vi "Apply Theme To UI Controls.vi"(8 "Error In":errorcluster, 11 "Appearance Actor in":refnum<class "Appearance Actor.lvclass">) -> (0 "Error Out":errorcluster, 3 "Appearance Actor out":refnum<class "Appearance Actor.lvclass">)   [LabVIEW 2021, in "Appearance Actor.lvlib" / "Appearance Actor.lvclass"]
uses:
  Appearance Actor.lvclass
  Appearance Actor.lvclass/Appearance Actor.ctl
  Theme Classes/Generic Theme/API/Typedefs/Window Element--enum.ctl
  Theme Classes/Generic Theme/Generic Theme.lvclass
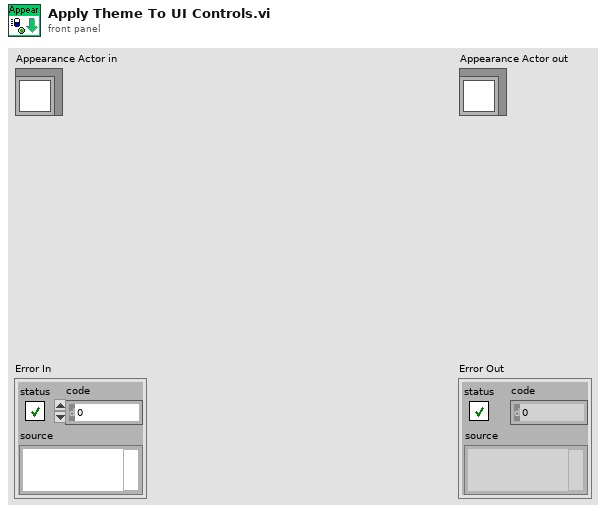
[diagram p1: front panel]
types:
  T1 = typedef "Appearance Actor.lvlib/Generic Theme.lvclass/Window Element--enum.ctl" = enum16{"None", "TB", "SM", "BP", "SB"}
  T2 = typedef "Appearance Actor.lvlib/Appearance Actor.lvclass/Control Reference Lists--cluster.ctl" = cluster{"TitleBar":T3, "SideMenu":T4, "BodyPane":T5, "StatusBar":T6}
  T3 = typedef "Appearance Actor.lvlib/Appearance Actor.lvclass/Control Reference Lists-TitleBar--cluster.ctl" = cluster{"Pane":refnum<vi>[], "Title":refnum<vi>, "Dark-CloseButton":refnum<vi>, "Light-CloseButton":refnum<vi>, "Dark-Buttons":refnum<vi>[], "Light-Buttons":refnum<vi>[], "Splitter":refnum<vi>}
  T4 = typedef "Appearance Actor.lvlib/Appearance Actor.lvclass/Control Reference Lists-SideMenu--cluster.ctl" = cluster{"Pane":refnum<vi>[], "Dark-Buttons":refnum<vi>[], "Light-Buttons":refnum<vi>[], "Splitter":refnum<vi>}
  T5 = typedef "Appearance Actor.lvlib/Appearance Actor.lvclass/Control Reference Lists-BodyPane--cluster.ctl" = cluster{"Pane":refnum<vi>[], "SubPanel":refnum<vi>}
  T6 = typedef "Appearance Actor.lvlib/Appearance Actor.lvclass/Control Reference Lists-StatusBar--cluster.ctl" = cluster{"Pane":refnum<vi>[], "Dark-Buttons":refnum<vi>[], "Light-Buttons":refnum<vi>[], "Splitter":refnum<vi>}
  T7 = typedef "Appearance Actor.lvlib/Generic Theme.lvclass/Theme Info--cluster.ctl" = cluster{"Name":string, "Type":string, "Version":string}
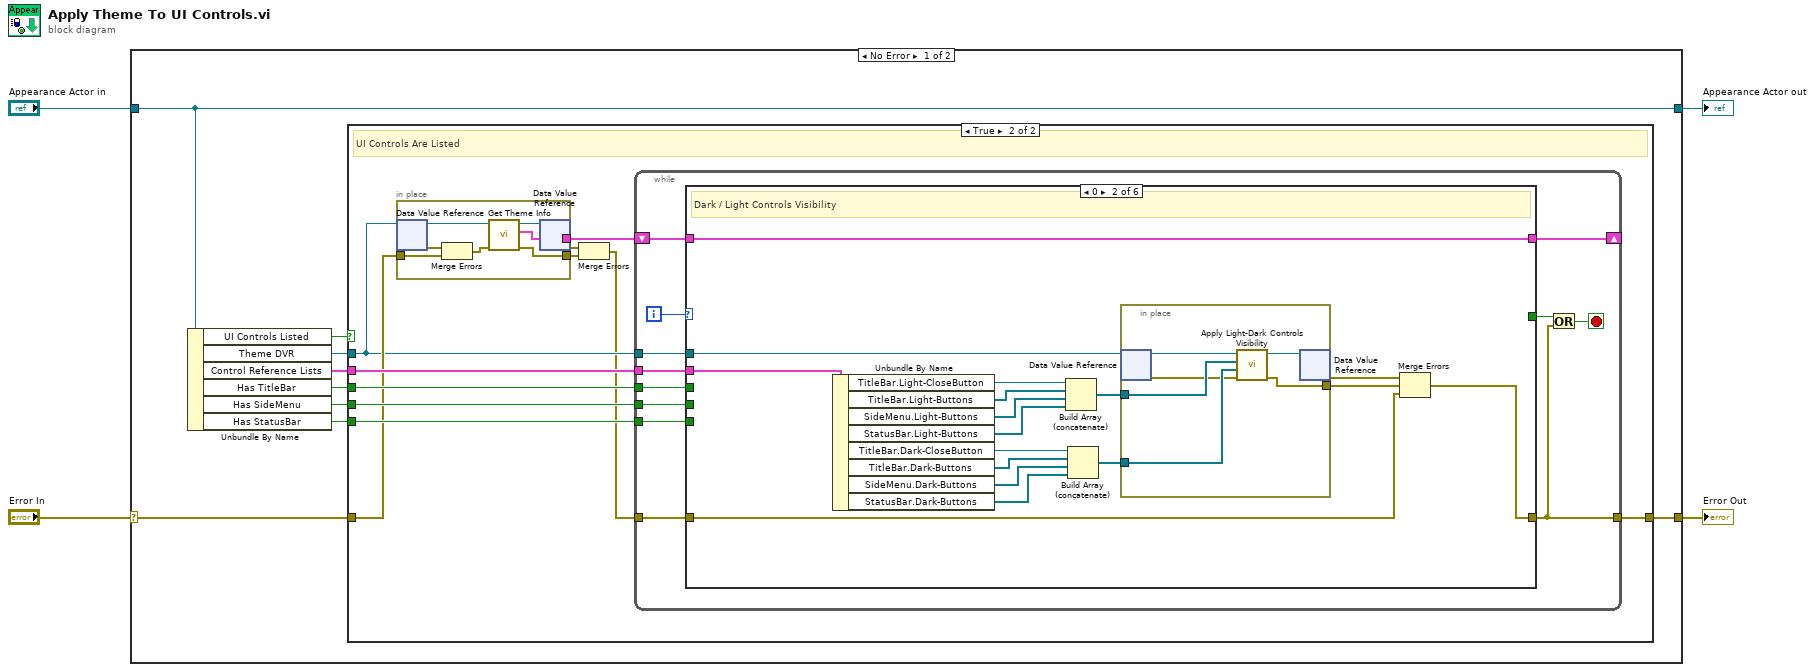
[diagram p0: block diagram]
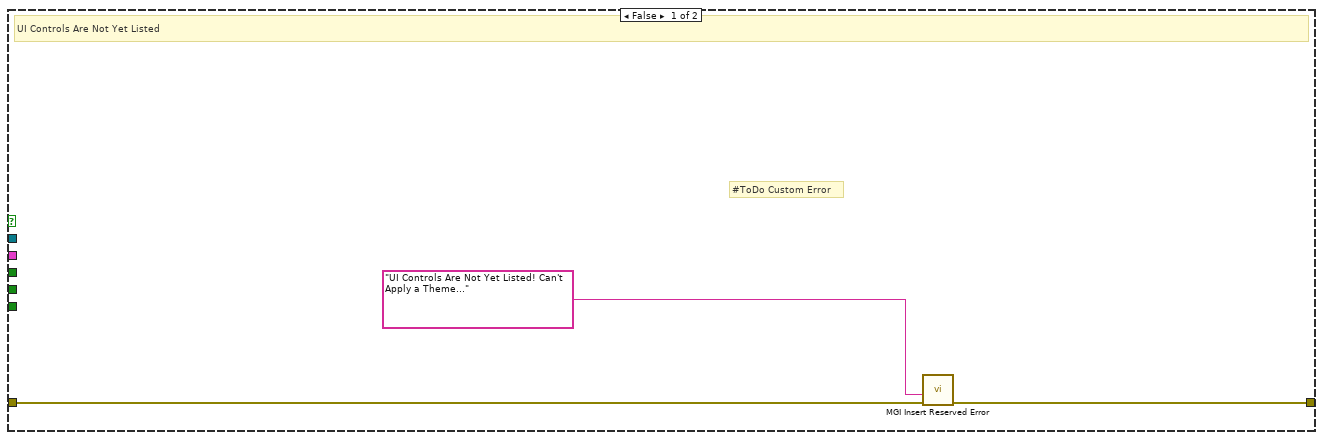
[diagram p2: hidden frame]
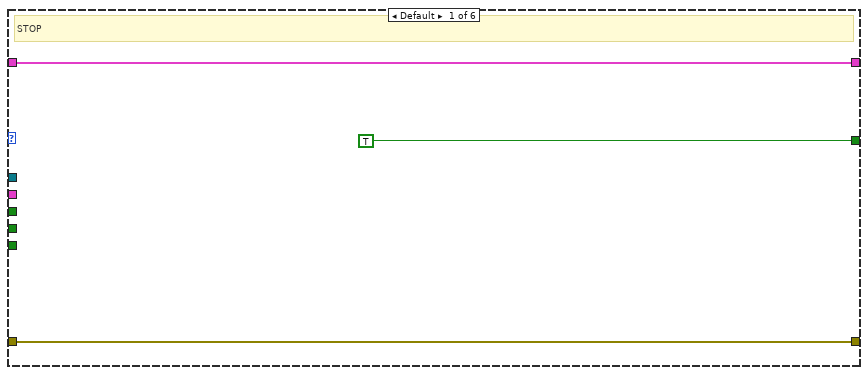
[diagram p3: hidden frame]
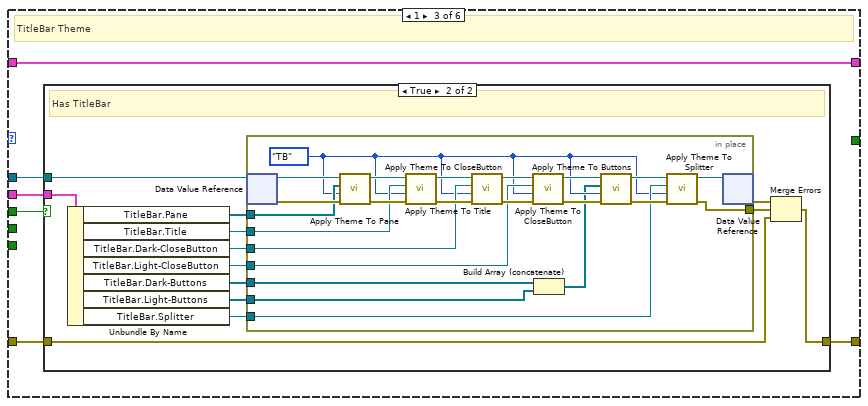
[diagram p4: hidden frame]
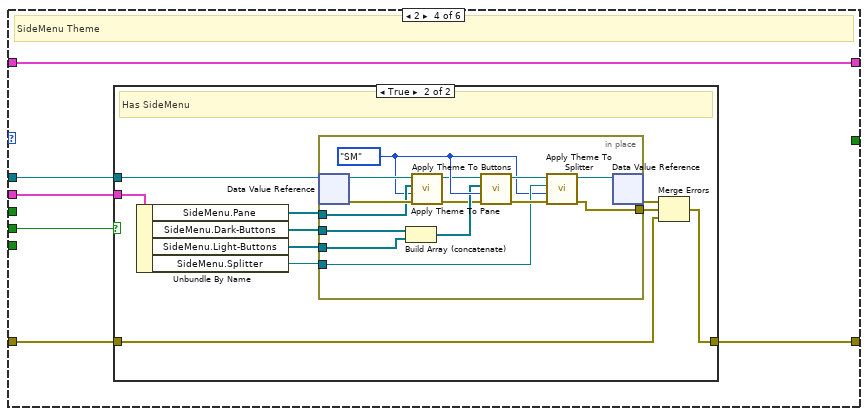
[diagram p6: hidden frame]
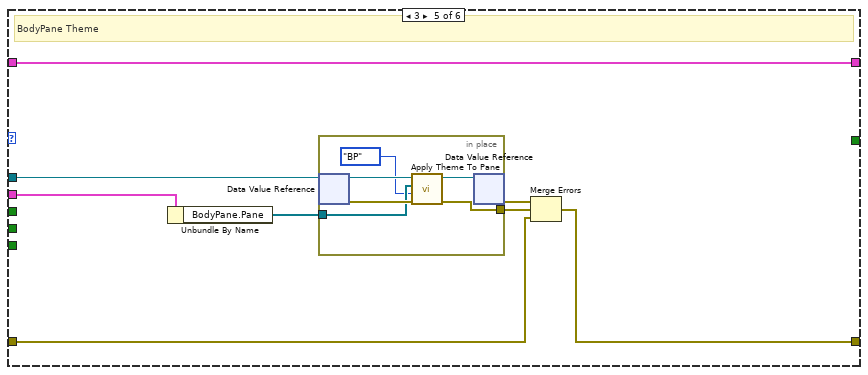
[diagram p8: hidden frame]
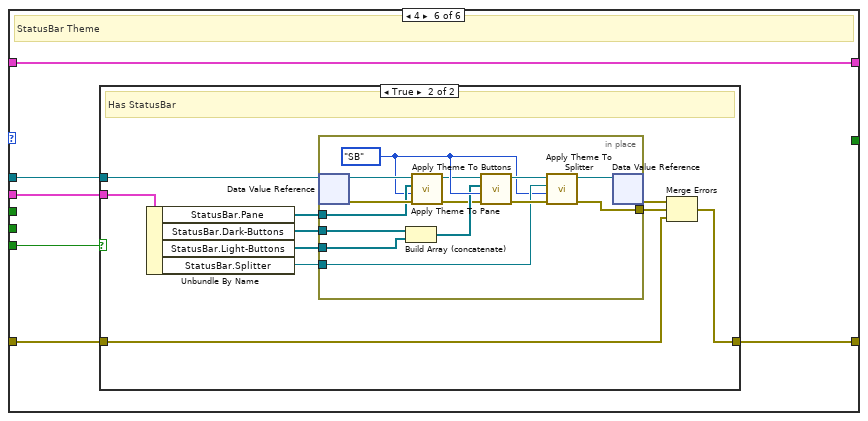
[diagram p9: hidden frame]
diagram:
  n1 = case shown="No Error" "Error In" {
    selector: "Error In" -> [w11 w193]
    tunnel: [w10 w193] -> w3
    tunnel: [w13 w192] -> w1
    tunnel: "Appearance Actor in" -> [w13 w192]
    frame No Error {
      n2 = Unbundle By Name(w13) -> ("UI Controls Listed"=w5:bool, "Theme DVR"=w12:refnum<data-value>, "Control Reference Lists"=w9:T2, "Has TitleBar"=w8:bool, "Has SideMenu"=w7:bool, "Has StatusBar"=w6:bool)
      n3 = case shown="True" w5 {
        tunnel: w12 -> [_ w20]
        tunnel: w11 -> [w16 w21]
        tunnel: [w15 w27] -> w10
        tunnel: w9 -> [_ w26]
        tunnel: w8 -> [_ w25]
        tunnel: w7 -> [_ w24]
        tunnel: w6 -> [_ w23]
        frame False {
          # "#ToDo Custom Error"
          # "UI Controls Are Not Yet Listed"
          n4 = call <userlib>:"MGI Insert Reserved Error.vi"("Error In"=w16, "Error Description"="UI Controls Are Not Yet Listed! Can't Apply a Theme..." ("format string")) -> ("Error Out"=w15:errorcluster)  [unwired: 9 in]
        }
        frame True {
          # "UI Controls Are Listed"
          n5 = in-place {
            in-place-border: [w34] -> w22
            in-place-border: w21 -> [w28]
            in-place-border: [w33] -> w17
            n6 = in-place-dvr #1(w20) -> (w32:refnum<class "Generic Theme.lvclass">, w30:errorcluster)
            n7 = Merge Errors(w30, w28) -> (w29:errorcluster)
            n8 = call-dynamic "Get Theme Info.vi"("Error In"=w29, "Generic Theme in"=w32) -> ("Error Out"=w33:errorcluster, "Theme Info"=w34:T7, "Generic Theme out"=w31:refnum<class "Generic Theme.lvclass">)  [unwired: 7 in]
            n9 = in-place-dvr #1(w31) -> (w18:errorcluster)  [unwired: 1 out]
          }
          n10 = Merge Errors(w18, w17) -> (w19:errorcluster)
          n11 = while {
            tunnel: w20 -> [w45]
            tunnel: w26 -> [w44]
            tunnel: w19 -> [w40]
            tunnel: [w41] -> w27
            tunnel: w25 -> [w39]
            tunnel: w24 -> [w38]
            tunnel: w23 -> [w37]
            shift-right: [w36] -> _
            shift-left: w22 -> [w35]
            i -> [w46]
            stop <- w42 stop-if-true
            n12 = case shown="0" w46 {
              tunnel: w45 -> [_ w52 w78 w121 w154 w166]
              tunnel: w44 -> [_ w63 w76 w118 w151 w164]
              tunnel: [TRUE _ _ _ _ _] -> w43
              tunnel: w40 -> [w48 w53 w74 w117 w148 w162]
              tunnel: [w48 w64 w77 w120 w152 w165] -> w41
              tunnel: w39 -> [_ _ w75 _ _ _]
              tunnel: w38 -> [_ _ _ w119 _ _]
              tunnel: w37 -> [_ _ _ _ _ w163]
              tunnel: [w47 w51 w73 w116 w147 w161] -> w36
              tunnel: w35 -> [w47 w51 w73 w116 w147 w161]
              frame Default {
                # "STOP"
              }
              frame 0 {
                # "Dark / Light Controls Visibility"
                n13 = Unbundle By Name(w63) -> ("TitleBar.Light-CloseButton"=w62:refnum<vi>, "TitleBar.Light-Buttons"=w61:refnum<vi>[], "SideMenu.Light-Buttons"=w60:refnum<vi>[], "StatusBar.Light-Buttons"=w59:refnum<vi>[], "TitleBar.Dark-CloseButton"=w58:refnum<vi>, "TitleBar.Dark-Buttons"=w57:refnum<vi>[], "SideMenu.Dark-Buttons"=w56:refnum<vi>[], "StatusBar.Dark-Buttons"=w55:refnum<vi>[])
                n14 = Build Array (concatenate)(w62, w61, w60, w59) -> (w50:refnum<vi>[])
                n15 = Build Array (concatenate)(w58, w57, w56, w55) -> (w54:refnum<vi>[])
                n16 = in-place {
                  in-place-border: [w71] -> w65
                  in-place-border: w50 -> [w70]
                  in-place-border: w54 -> [w69]
                  n17 = in-place-dvr #2(w52) -> (w68:refnum<class "Generic Theme.lvclass">, w67:errorcluster)
                  n18 = call-dynamic "Apply Light-Dark Controls Visibility.vi"("Error In"=w67, "Dark Controls"=w69, "Light Controls"=w70, "Generic Theme in"=w68) -> ("Error Out"=w71:errorcluster, "Generic Theme out"=w72:refnum<class "Generic Theme.lvclass">)  [unwired: 6 in]
                  n19 = in-place-dvr #2(w72) -> (w66:errorcluster)  [unwired: 1 out]
                }
                n20 = Merge Errors(w66, w65, w53) -> (w64:errorcluster)
              }
              frame 1 {
                # "TitleBar Theme"
                n21 = case shown="True" w75 {
                  tunnel: w78 -> [_ w92]
                  tunnel: [w79 w89] -> w77
                  tunnel: w76 -> [_ w88]
                  tunnel: w74 -> [w79 w80]
                  frame False {
                    # "No TitleBar"
                  }
                  frame True {
                    # "Has TitleBar"
                    n22 = Unbundle By Name(w88) -> ("TitleBar.Pane"=w87:refnum<vi>[], "TitleBar.Title"=w86:refnum<vi>, "TitleBar.Dark-CloseButton"=w85:refnum<vi>, "TitleBar.Light-CloseButton"=w82:refnum<vi>, "TitleBar.Dark-Buttons"=w84:refnum<vi>[], "TitleBar.Light-Buttons"=w81:refnum<vi>[], "TitleBar.Splitter"=w83:refnum<vi>)
                    n23 = in-place {
                      in-place-border: [w107] -> w90
                      in-place-border: w87 -> [w105]
                      in-place-border: w86 -> [w104]
                      in-place-border: w85 -> [w103]
                      in-place-border: w84 -> [w95]
                      in-place-border: w83 -> [w102]
                      in-place-border: w82 -> [w97]
                      in-place-border: w81 -> [w94]
                      w96 = Window_Element--enum."TB" ("Window Element")
                      n24 = in-place-dvr #3(w92) -> (w115:refnum<class "Generic Theme.lvclass">, w114:errorcluster)
                      n25 = call-dynamic "Apply Theme To Pane.vi"("Error In"=w114, "Window Element"=w96, "Pane Refs"=w105, "Generic Theme in"=w115) -> ("Error Out"=w110:errorcluster, "Generic Theme out"=w113:refnum<class "Generic Theme.lvclass">)  [unwired: 6 in]
                      n26 = call-dynamic "Apply Theme To Title.vi"("Error In"=w110, "Window Element"=w96, "Title Ref"=w104, "Generic Theme in"=w113) -> ("Error Out"=w109:errorcluster, "Generic Theme out"=w112:refnum<class "Generic Theme.lvclass">)  [unwired: 6 in]
                      n27 = call-dynamic "Apply Theme To CloseButton.vi"("Error In"=w109, "Window Element"=w96, "CloseButton Ref"=w103, "Generic Theme in"=w112) -> ("Error Out"=w101:errorcluster, "Generic Theme out"=w100:refnum<class "Generic Theme.lvclass">)  [unwired: 6 in]
                      n28 = call-dynamic "Apply Theme To CloseButton.vi"("Error In"=w101, "Window Element"=w96, "CloseButton Ref"=w97, "Generic Theme in"=w100) -> ("Error Out"=w98:errorcluster, "Generic Theme out"=w99:refnum<class "Generic Theme.lvclass">)  [unwired: 6 in]
                      n29 = Build Array (concatenate)(w95, w94) -> (w93:refnum<vi>[])
                      n30 = call-dynamic "Apply Theme To Buttons.vi"("Error In"=w98, "Window Element"=w96, "Buttons Ref"=w93, "Generic Theme in"=w99) -> ("Error Out"=w108:errorcluster, "Generic Theme out"=w111:refnum<class "Generic Theme.lvclass">)  [unwired: 6 in]
                      n31 = call-dynamic "Apply Theme To Splitter.vi"("Error In"=w108, "Window Element"=w96, "Splitter Ref"=w102, "Generic Theme in"=w111) -> ("Error Out"=w107:errorcluster, "Generic Theme out"=w106:refnum<class "Generic Theme.lvclass">)  [unwired: 6 in]
                      n32 = in-place-dvr #3(w106) -> (w91:errorcluster)  [unwired: 1 out]
                    }
                    n33 = Merge Errors(w91, w90, w80) -> (w89:errorcluster)
                  }
                }
              }
              frame 2 {
                # "SideMenu Theme"
                n34 = case shown="True" w119 {
                  tunnel: w121 -> [_ w132]
                  tunnel: [w122 w129] -> w120
                  tunnel: w118 -> [_ w128]
                  tunnel: w117 -> [w122 w123]
                  frame False {
                    # "No SideMenu"
                  }
                  frame True {
                    # "Has SideMenu"
                    n35 = Unbundle By Name(w128) -> ("SideMenu.Pane"=w127:refnum<vi>[], "SideMenu.Dark-Buttons"=w126:refnum<vi>[], "SideMenu.Light-Buttons"=w125:refnum<vi>[], "SideMenu.Splitter"=w124:refnum<vi>)
                    n36 = in-place {
                      in-place-border: [w133] -> w130
                      in-place-border: w127 -> [w141]
                      in-place-border: w126 -> [w138]
                      in-place-border: w124 -> [w140]
                      in-place-border: w125 -> [w137]
                      w139 = Window_Element--enum."SM" ("Window Element")
                      n37 = in-place-dvr #4(w132) -> (w146:refnum<class "Generic Theme.lvclass">, w145:errorcluster)
                      n38 = Build Array (concatenate)(w138, w137) -> (w136:refnum<vi>[])
                      n39 = call-dynamic "Apply Theme To Pane.vi"("Error In"=w145, "Window Element"=w139, "Pane Refs"=w141, "Generic Theme in"=w146) -> ("Error Out"=w134:errorcluster, "Generic Theme out"=w135:refnum<class "Generic Theme.lvclass">)  [unwired: 6 in]
                      n40 = call-dynamic "Apply Theme To Buttons.vi"("Error In"=w134, "Window Element"=w139, "Buttons Ref"=w136, "Generic Theme in"=w135) -> ("Error Out"=w143:errorcluster, "Generic Theme out"=w144:refnum<class "Generic Theme.lvclass">)  [unwired: 6 in]
                      n41 = call-dynamic "Apply Theme To Splitter.vi"("Error In"=w143, "Window Element"=w139, "Splitter Ref"=w140, "Generic Theme in"=w144) -> ("Error Out"=w133:errorcluster, "Generic Theme out"=w142:refnum<class "Generic Theme.lvclass">)  [unwired: 6 in]
                      n42 = in-place-dvr #4(w142) -> (w131:errorcluster)  [unwired: 1 out]
                    }
                    n43 = Merge Errors(w131, w130, w123) -> (w129:errorcluster)
                  }
                }
              }
              frame 3 {
                # "BodyPane Theme"
                n44 = Unbundle By Name(w151) -> ("BodyPane.Pane"=w150:refnum<vi>[])
                n45 = in-place {
                  in-place-border: w150 -> [w158]
                  in-place-border: [w155] -> w149
                  n46 = in-place-dvr #5(w154) -> (w160:refnum<class "Generic Theme.lvclass">, w159:errorcluster)
                  n47 = call-dynamic "Apply Theme To Pane.vi"("Error In"=w159, "Window Element"=Window_Element--enum."BP", "Pane Refs"=w158, "Generic Theme in"=w160) -> ("Error Out"=w155:errorcluster, "Generic Theme out"=w156:refnum<class "Generic Theme.lvclass">)  [unwired: 6 in]
                  n48 = in-place-dvr #5(w156) -> (w153:errorcluster)  [unwired: 1 out]
                }
                n49 = Merge Errors(w153, w149, w148) -> (w152:errorcluster)
              }
              frame 4 {
                # "StatusBar Theme"
                n50 = case shown="True" w163 {
                  tunnel: w166 -> [_ w177]
                  tunnel: [w167 w175] -> w165
                  tunnel: w164 -> [_ w174]
                  tunnel: w162 -> [w167 w168]
                  frame False {
                    # "No StatusBar"
                  }
                  frame True {
                    # "Has StatusBar"
                    n51 = Unbundle By Name(w174) -> ("StatusBar.Pane"=w173:refnum<vi>[], "StatusBar.Dark-Buttons"=w172:refnum<vi>[], "StatusBar.Light-Buttons"=w170:refnum<vi>[], "StatusBar.Splitter"=w171:refnum<vi>)
                    n52 = in-place {
                      in-place-border: w173 -> [w186]
                      in-place-border: w172 -> [w183]
                      in-place-border: w171 -> [w185]
                      in-place-border: w170 -> [w182]
                      in-place-border: [w178] -> w169
                      w184 = Window_Element--enum."SB" ("Window Element")
                      n53 = in-place-dvr #6(w177) -> (w191:refnum<class "Generic Theme.lvclass">, w190:errorcluster)
                      n54 = Build Array (concatenate)(w183, w182) -> (w181:refnum<vi>[])
                      n55 = call-dynamic "Apply Theme To Pane.vi"("Error In"=w190, "Window Element"=w184, "Pane Refs"=w186, "Generic Theme in"=w191) -> ("Error Out"=w179:errorcluster, "Generic Theme out"=w180:refnum<class "Generic Theme.lvclass">)  [unwired: 6 in]
                      n56 = call-dynamic "Apply Theme To Buttons.vi"("Error In"=w179, "Window Element"=w184, "Buttons Ref"=w181, "Generic Theme in"=w180) -> ("Error Out"=w188:errorcluster, "Generic Theme out"=w189:refnum<class "Generic Theme.lvclass">)  [unwired: 6 in]
                      n57 = call-dynamic "Apply Theme To Splitter.vi"("Error In"=w188, "Window Element"=w184, "Splitter Ref"=w185, "Generic Theme in"=w189) -> ("Error Out"=w178:errorcluster, "Generic Theme out"=w187:refnum<class "Generic Theme.lvclass">)  [unwired: 6 in]
                      n58 = in-place-dvr #6(w187) -> (w176:errorcluster)  [unwired: 1 out]
                    }
                    n59 = Merge Errors(w176, w169, w168) -> (w175:errorcluster)
                  }
                }
              }
            }
            n60 = Or(x=w43, y=w41) -> (x .or. y?=w42:bool)
          }
        }
      }
    }
    frame Error {
    }
  }
  "Error Out" <- w3
  "Appearance Actor out" <- w1
